vi "Process.vi"(11 "Actor":refnum<class "Info View.lvclass">) -> ()   [LabVIEW 2015, in "Info View.lvclass"]
uses:
  Info View.lvclass
  Re-use Libraries/Utility/UI/System Button (without mouse hover).ctl
  Re-use Libraries/Minimal Actor Framework/Actors/Base Actor/Actor/Front Panel State.ctl
  Actors/Main Controller/Actor/Windows.ctl
  Globals.vi
  Actors/Main Controller/API/Main Controller Actor API.lvclass
  Re-use Libraries/Minimal Actor Framework/Actors/Base Actor/Actor/Actor.lvclass
  Re-use Libraries/Minimal Actor Framework/Messaging/Message/Message.lvclass
  Actors/Alarm Handler/API/Alarm Handler Actor API.lvclass
  Re-use Libraries/Application Info/App Info.lvlib
  Actors/Main Controller/Actor/Main Controller Actor.lvclass
  Re-use Libraries/Utility/Utility.lvlib
panel:
  in  "About":T1
  out "Application Version":string
  out "Application Name":string
  in  "Minimise":T1
  in  "Shutdown Application":T1
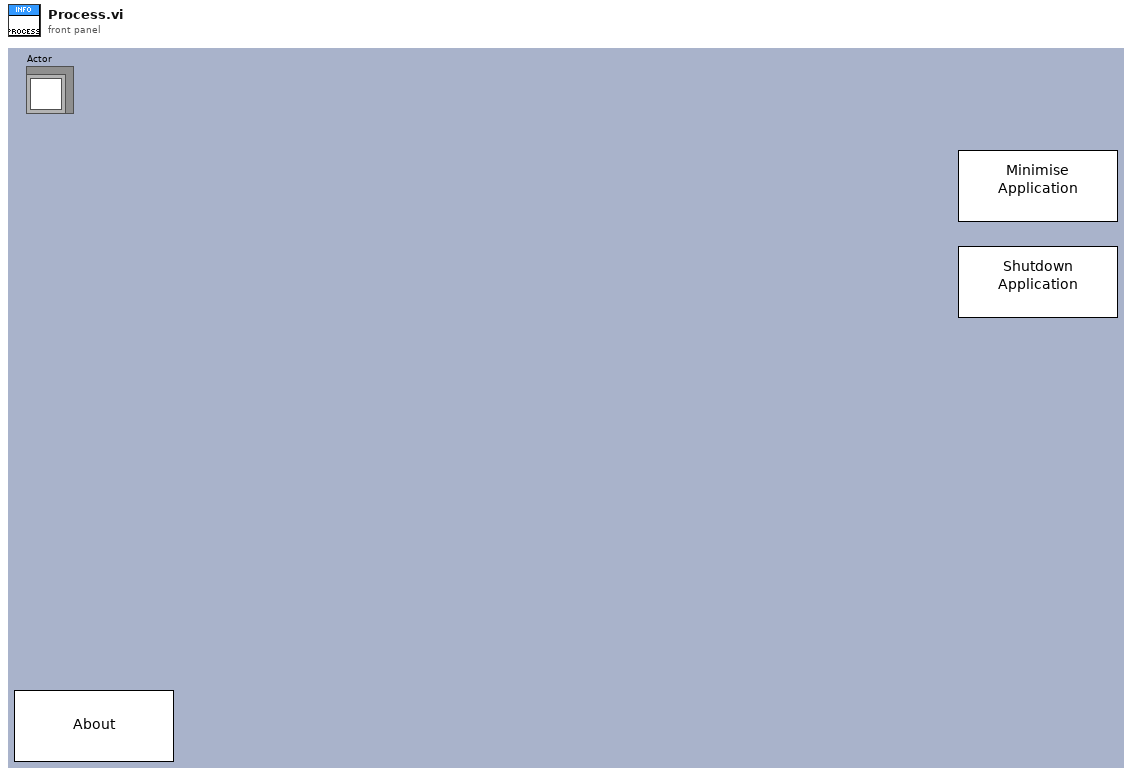
[diagram p1: front panel]
types:
  T1 = typedef "Utility.lvlib/System Button (without mouse hover).ctl" = bool
  T2 = typedef "Actor.lvclass/Front Panel State.ctl" = enum32{"Invalid", "Standard", "Closed", "Hidden", "Minimized", "Maximized"}
  T3 = typedef "Main Controller Actor.lvclass/Windows.ctl" = enum16{"About", "Status", "Debugger"}
  T4 = typedef "App Info.lvlib/Core Data.ctl" = cluster{"Version":string, "Misc Info":string, "Name":string, "Name 2":string}
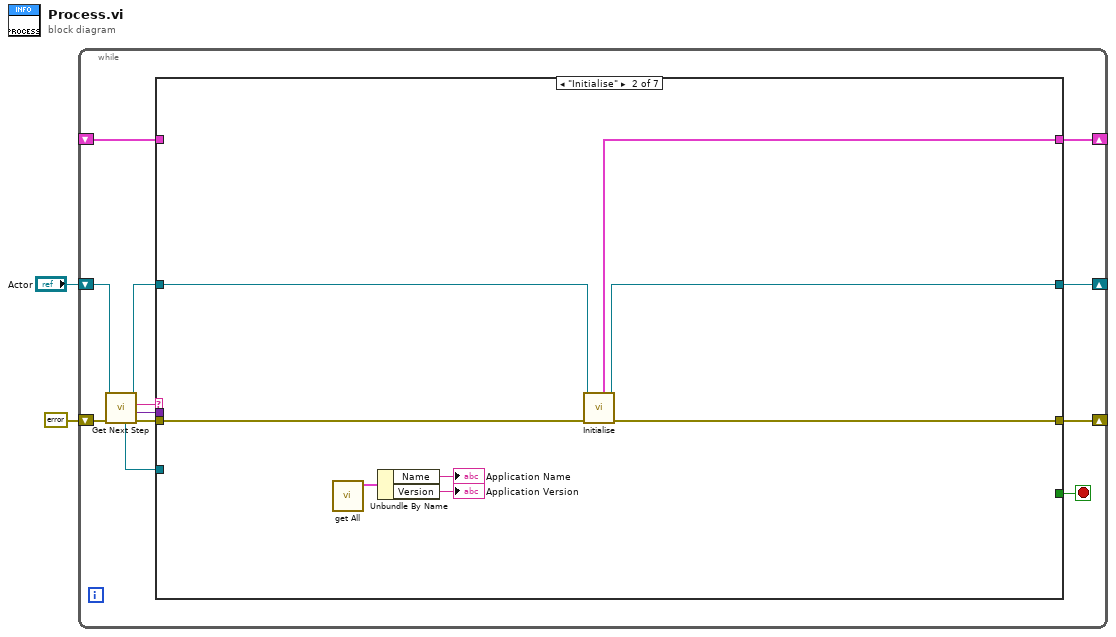
[diagram p0: block diagram]
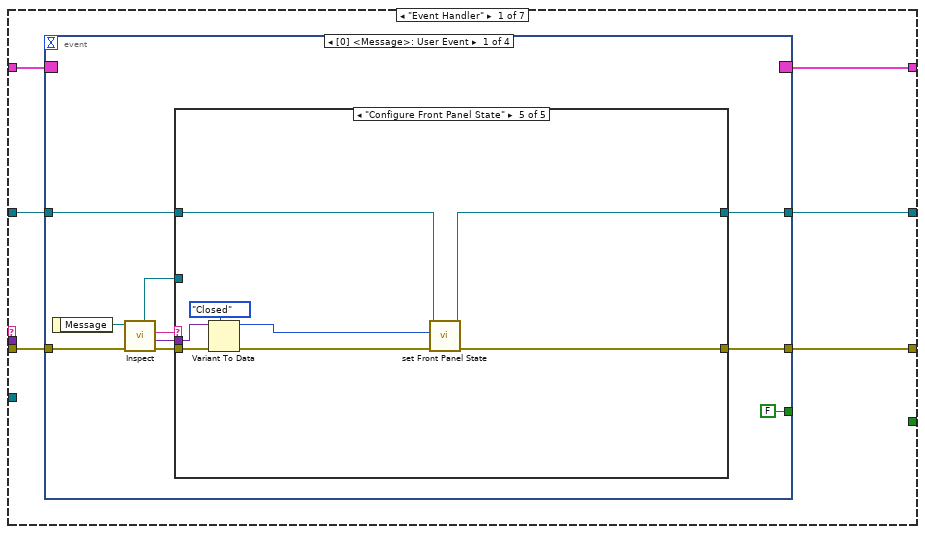
[diagram p2: hidden frame]
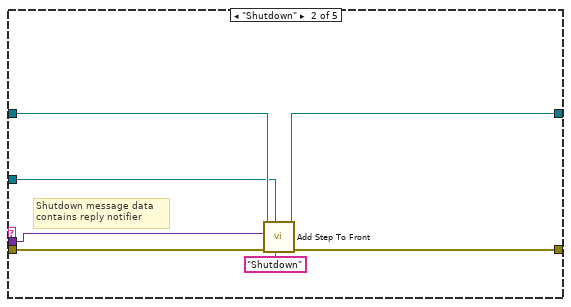
[diagram p4: hidden frame]
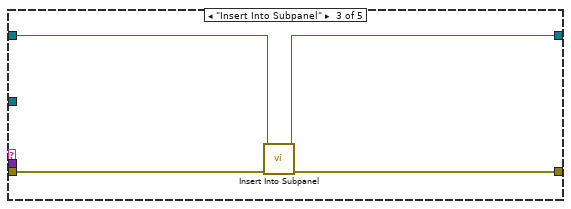
[diagram p5: hidden frame]
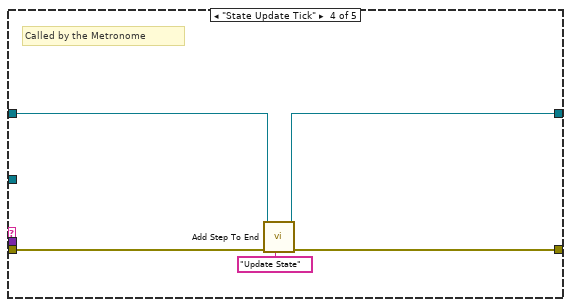
[diagram p6: hidden frame]
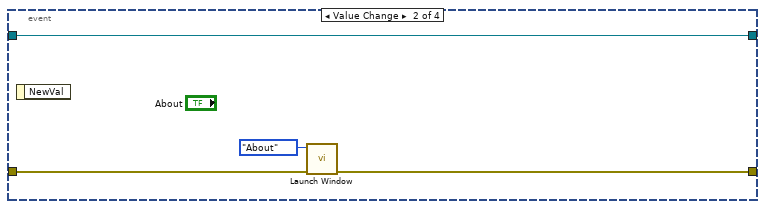
[diagram p7: hidden frame]
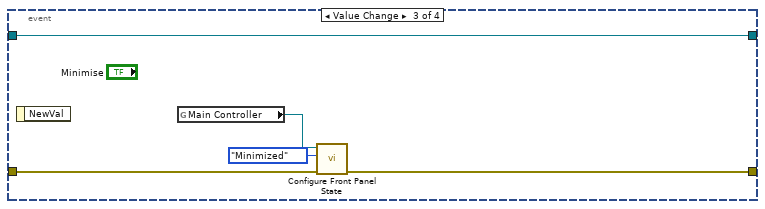
[diagram p8: hidden frame]
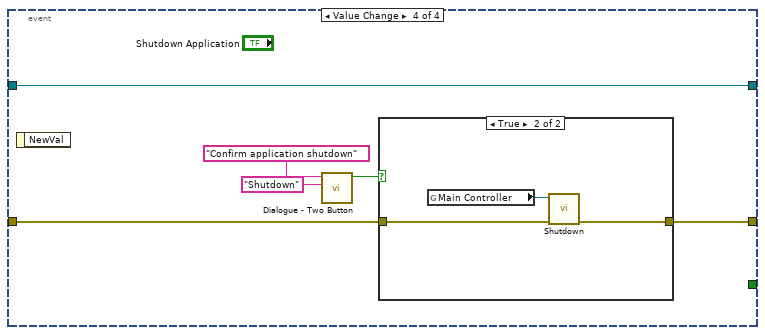
[diagram p9: hidden frame]
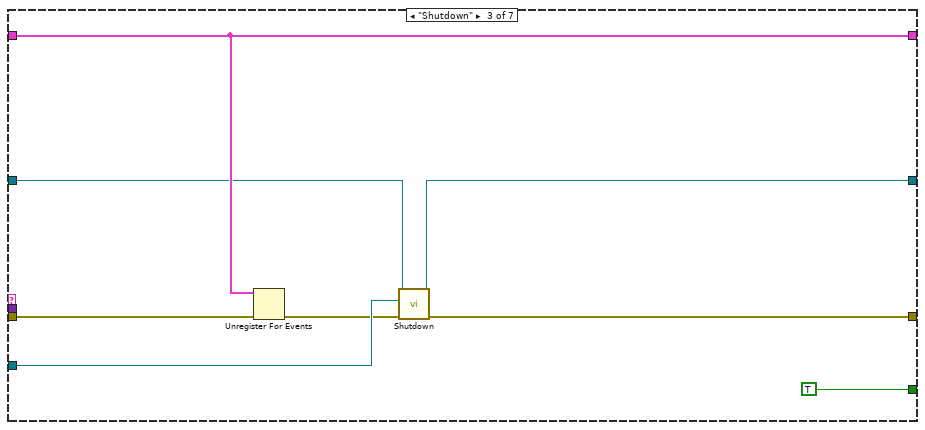
[diagram p11: hidden frame]
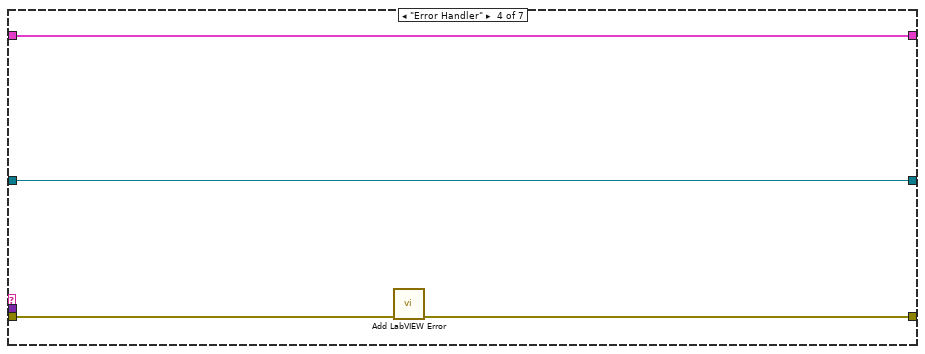
[diagram p12: hidden frame]
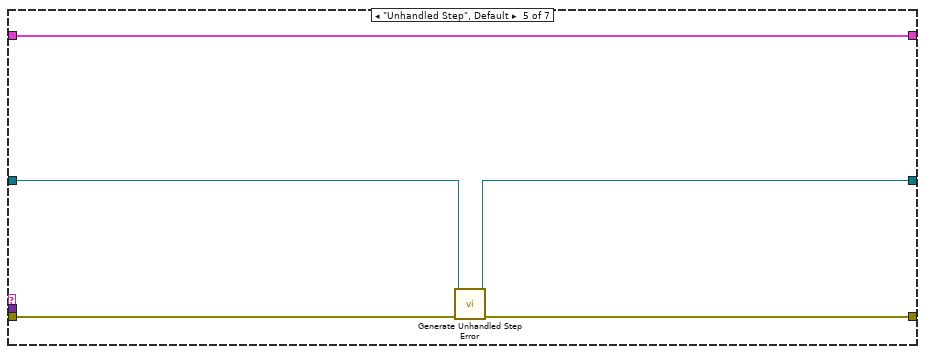
[diagram p13: hidden frame]
diagram:
  n1 = while {
    shift-right: [w5] -> _
    shift-left: "Actor" -> [w13]
    shift-right: [w10] -> _
    shift-left: _ -> [w9]
    shift-right: [w4] -> _
    shift-left: errorcluster {"status"=FALSE, "code"=0, "source"=""} ("error constant") -> [w7]
    stop <- w14 stop-if-true
    n2 = call-dynamic "Get Next Step.vi"("error in (no error)"=w7, "Actor in"=w13) -> ("error out"=w8:errorcluster, "Parameter"=w11:variant, "Step"=w6:string, "Actor out"=w12:refnum<class "Info View.lvclass">, "Reply Channel"=w3:refnum<notifier>)  [unwired: 5 in]
    n3 = case shown="\"Initialise\"" w6 {
      tunnel: [_ _ TRUE _ _ _ _] -> w14
      tunnel: w12 -> [w20 w81 w89 w92 w99 w102 w104]
      tunnel: [w19 w76 w88 w92 w98 w102 w104] -> w5
      tunnel: w11 -> [_ _ _ _ _ _ _]
      tunnel: [w17 w83 w90 w95 w100 w103 w106] -> w10
      tunnel: w9 -> [w18 _ w90 w95 w100 w103 w106]
      tunnel: w8 -> [w16 w80 w86 w94 w97 w101 w105]
      tunnel: [w15 w82 w84 w93 w96 w101 w105] -> w4
      tunnel: w3 -> [_ _ w87 _ _ _ _]
      frame "Event Handler" {
        n4 = event shown="[0] <Message>: User Event" {
          selector: w18 -> [_ _ _ _]
          dyn-events: [_ _ _ _] -> w17
          timeout: _ -> [_ _ _ _]
          tunnel: w20 -> [w30 w60 w65 w71]
          tunnel: [w29 w60 w65 w71] -> w19
          tunnel: w16 -> [w27 w59 w64 w67]
          tunnel: [w28 w58 w63 w66] -> w15
          tunnel: [FALSE _ _ _] -> _
          event User Event {
            n5 = event-data() -> ("Message"=w26:refnum<class "Message.lvclass">)  [unwired: 1 in]
            n6 = call "Inspect.vi"("error in (no error)"=w27, "Message in"=w26) -> ("error out"=w23:errorcluster, "Data"=w24:variant, "Name"=w25:string, "Reply Channel"=w22:refnum<notifier>)  [unwired: 5 in, 1 out]
            n7 = case shown="\"Configure Front Panel State\"" w25 {
              tunnel: w30 -> [w32 w39 w43 w48 w56]
              tunnel: [w32 w38 w42 w47 w55] -> w29
              tunnel: w23 -> [w31 w36 w41 w45 w52]
              tunnel: [w31 w35 w40 w44 w54] -> w28
              tunnel: w24 -> [_ w34 _ _ w53]
              tunnel: w22 -> [_ w33 _ _ _]
              frame Default {
              }
              frame "Shutdown" {
                # "Shutdown message data contains reply notifier"
                n8 = call-dynamic "Add Step To Front.vi"("Step Name"="Shutdown", "Reply Channel"=w33, "error in (no error)"=w36, "Parameter"=w34, "Actor in"=w39) -> ("error out"=w35:errorcluster, "Actor out"=w38:refnum<class "Info View.lvclass">)  [unwired: 5 in]
              }
              frame "Insert Into Subpanel" {
                n9 = call-dynamic "Insert Into Subpanel.vi"("error in (no error)"=w41, "Actor in"=w43) -> ("error out"=w40:errorcluster, "Actor out"=w42:refnum<class "Info View.lvclass">)  [unwired: 8 in]
              }
              frame "State Update Tick" {
                # "Called by the Metronome"
                n10 = call-dynamic "Add Step To End.vi"("Step Name"="Update State", "error in (no error)"=w45, "Actor in"=w48) -> ("error out"=w44:errorcluster, "Actor out"=w47:refnum<class "Info View.lvclass">)  [unwired: 7 in]
              }
              frame "Configure Front Panel State" {
                n11 = Variant To Data(error in=w52, type=Front_Panel_State."Closed" ("Front Panel State"), Variant=w53) -> (data=w49:T2, error out=w51:errorcluster)
                n12 = call-dynamic "set Front Panel State.vi"("error in (no error)"=w51, "Front Panel State"=w49, "Actor in"=w56) -> ("error out"=w54:errorcluster, "Actor out"=w55:refnum<class "Info View.lvclass">)  [unwired: 7 in]
              }
            }
          }
          event Value Change {
            n13 = event-data() -> ()  [unwired: 1 in, 1 out]
            n14 = call "Launch Window.vi"("error in (no error)"=w59, "Window"=Windows."About") -> ("error out"=w58:errorcluster)  [unwired: 9 in]
          }
          event Value Change {
            n15 = event-data() -> ()  [unwired: 1 in, 1 out]
            n16 = global read "Globals.vi" "Main Controller"() -> (w62:refnum<class "Main Controller Actor API.lvclass">)
            n17 = call-dynamic "Configure Front Panel State.vi"("error in (no error)"=w64, "Front Panel State"=Front_Panel_State."Minimized", "Actor API in"=w62) -> ("error out"=w63:errorcluster)  [unwired: 8 in]
          }
          event Value Change {
            n18 = event-data() -> ()  [unwired: 1 in, 1 out]
            n19 = call "Dialogue - Two Button.vi"("True Button Text"="Shutdown" ("T button name (\"OK\")"), "Message"="Confirm application shutdown" ("message")) -> ("True Button Pressed"=w70:bool)  [unwired: 9 in]
            n20 = case shown="True" w70 {
              tunnel: w67 -> [w72 w74]
              tunnel: [w72 w73] -> w66
              frame False {
              }
              frame True {
                n21 = global read "Globals.vi" "Main Controller"() -> (w75:refnum<class "Main Controller Actor API.lvclass">)
                n22 = call-dynamic "Shutdown.vi"("error in (no error)"=w74, "Actor API in"=w75) -> ("error out"=w73:errorcluster)  [unwired: 9 in]
              }
            }
          }
        }
      }
      frame "Initialise" {
        n23 = call "get All.vi"() -> ("Data out"=w78:T4)  [unwired: 10 in, 1 out]
        n24 = Unbundle By Name(w78) -> ("Name"=→"Application Name":string, "Version"=→"Application Version":string)
        n25 = call "Initialise.vi"("error in (no error)"=w80, "Actor in"=w81) -> ("error out"=w82:errorcluster, "Actor out"=w76:refnum<class "Info View.lvclass">, "Observers"=w83:cluster{"Actor":refnum<event-registration>})  [unwired: 7 in]
      }
      frame "Shutdown" {
        n26 = Unregister For Events(event registration refnum=w90, error in=w86) -> (error out=w85:errorcluster)
        n27 = call-dynamic "Shutdown.vi"("error in (no error)"=w85, "Reply Channel"=w87, "Actor in"=w89) -> ("error out"=w84:errorcluster, "Actor out"=w88:refnum<class "Info View.lvclass">)  [unwired: 7 in]
      }
      frame "Error Handler" {
        n28 = call "Add LabVIEW Error.vi"("error in (no error)"=w94) -> ("error out"=w93:errorcluster)  [unwired: 10 in]
      }
      frame "Unhandled Step", Default {
        n29 = call-dynamic "Generate Unhandled Step Error.vi"("error in (no error)"=w97, "Actor in"=w99) -> ("error out"=w96:errorcluster, "Actor out"=w98:refnum<class "Info View.lvclass">)  [unwired: 8 in]
      }
      frame "-----------------------" {
        # "Separator"
      }
      frame "Update State" {
        # "Not used"
      }
    }
  }
